vi "Get Owning Task.vi"(8 "error in (no error)":errorcluster, 11 "Group in":refnum<class "Group.lvclass">) -> (0 "error out":errorcluster, 2 "Task":string, 3 "Group out":refnum<class "Group.lvclass">)   [LabVIEW 2020, in "Vecto.lvlib" / "Group.lvclass"]
uses:
  Group.lvclass
  Group Config/Group Config.lvclass
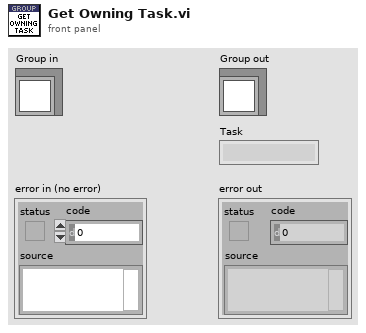
[diagram p1: front panel]
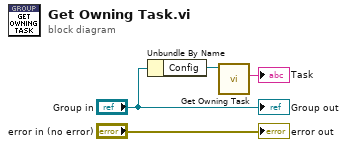
[diagram p0: block diagram]
diagram:
  n1 = Unbundle By Name("Group in") -> ("Config"=w2:refnum<class "Group Config.lvclass">)
  n2 = call "Get Owning Task.vi"("Group Config in"=w2) -> ("Task"=→"Task":string)  [unwired: 8 in, 2 out]
  "error out" <- "error in (no error)"
  "Group out" <- "Group in"
